vi "Day 6.vi"() -> ()   [LabVIEW 2020]
uses:
  3fa8e623-7fc4-4fee-bd88-71eac602b765.vi
  8efd2a67-bb32-401c-9d86-5bcad490fe8b.vi
panel:
  out "Solution":i32
  out "Solution":i32
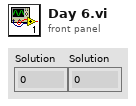
[diagram p1: front panel]
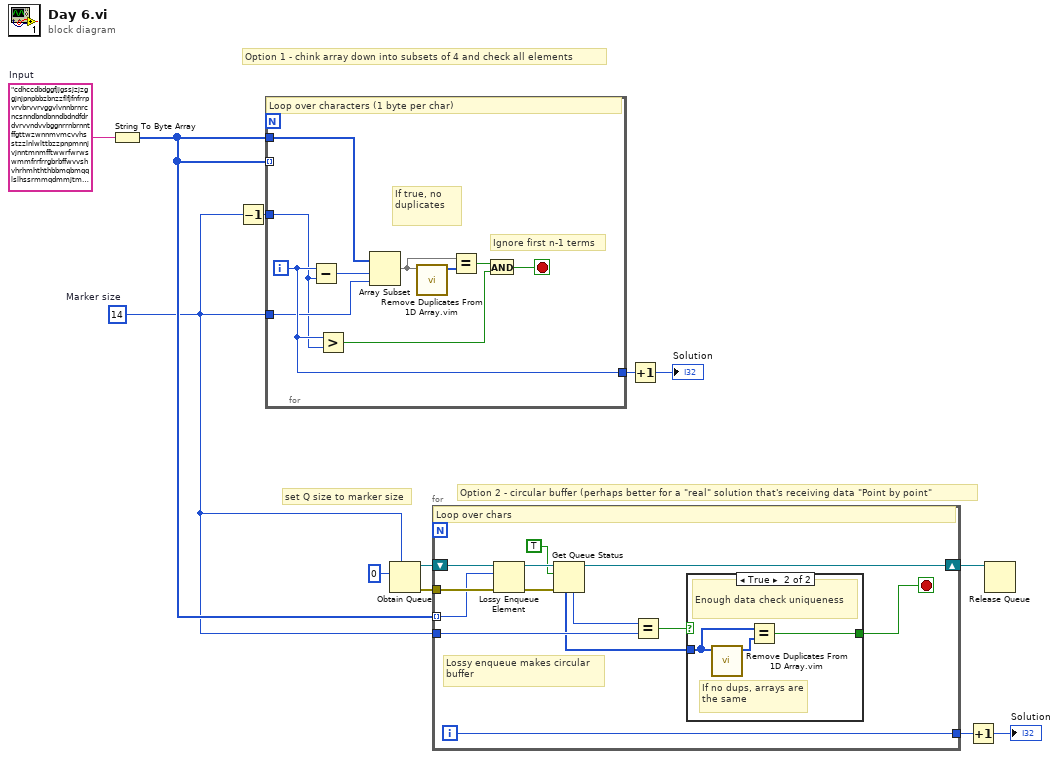
[diagram p0: block diagram]
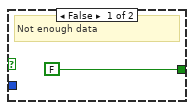
[diagram p2: hidden frame]
diagram:
  w5 = 14  # Marker size
  w9 = "cdhccdbdggfjjgssjzjzggjnjpnpbbzbnzzflfjfnfrrpvrvbrvvrvggvlvnnbrnrcncsnndbndbnndbdndfdrdvrvvndvvbggnrrnbrnntffgttwzwnnmvmcvvhsstzzlnlwlttbzzpnpmnnjvjnntmnmfftwwrfwrwswmmfrrfrrgbrbffwvvshvhrhmhththbbmqbmqqlslhssrmmqdmmjtmtmjtmjtttnwnvwvqwqjjnbbbdbqbnbpnbnllglcglcgcdczdznnqhhfthtmtlldqlqrrmddrldlzdllvddjcddqfqbqsbqqnllwppqpqzzrbbdppzsppjdpdqpdqdfqfrrwbwrwwqcqcsqsvvpbvbbztzptzzpccdtdhdffvqvcvzzmwzwddjfdffplplqlvlmmmvggpmpvpddpbptplpvlplvpvvnrvnnbqqqjhhwfhwfhwhqhmmpphqpqvppfzpzjzddgzzwffjmjggwhwwnnmlmpmmhcmcpcrcddvzvpzzwnznfznffgdgvddvtvgvsvdsdbbjnjtntbnttgbbbvgvgrgrzrvzrzddlsddcndcnnfqnnmpmlppdlpl..."  # Input
  # "Option 2 - circular buffer (perhaps better for a \"real\" solution that's receiving data \"Point by point\""
  # "Option 1 - chink array down into subsets of 4 and check all elements"
  # "set Q size to marker size"
  n1 = String To Byte Array(string=w9) -> (unsigned byte array=w8:u8[])
  n2 = Decrement(x=w5) -> (x-1=w10:i32)
  n3 = for {
    tunnel: w8 -> [w22]
    tunnel: [w20] -> w12
    tunnel: w5 -> [w17]
    tunnel: w10 -> [w16]
    tunnel: w8 -> [_] mode=indexing
    i -> [w20]
    stop <- w18 stop-if-true
    # "Ignore first n-1 terms"
    # "If true, no duplicates"
    # "Loop over characters (1 byte per char)"
    n4 = Subtract(x=w20, y=w16) -> (x-y=w21:i32)
    n5 = Greater?(x=w20, y=w16) -> (0:w19:bool)
    n6 = Array Subset(array=w22, index=w21, length=w17) -> (w14:u8[])
    n7 = call "Remove Duplicates From 1D Array.vim"("array"=w14) -> ("array with duplicates removed"=w15:u8[])  [unwired: 10 in]
    n8 = Equal?(x=w14, y=w15) -> (x = y?=w13:bool)
    n9 = And(x=w13, y=w19) -> (x .and. y?=w18:bool)
  }
  n10 = Obtain Queue(max queue size (-1, unlimited)=w5, element data type=u8 0) -> (queue out=w6:refnum<queue>, error out=w7:errorcluster)  [unwired: 3 in, 1 out]
  n11 = for {
    tunnel: w8 -> [w33] mode=indexing
    tunnel: w7 -> [w35]
    tunnel: w5 -> [w29]
    tunnel: [w24] -> w4
    shift-right: [w23] -> w1
    shift-left: w6 -> [w34]
    i -> [w24]
    stop <- w25 stop-if-true
    # "Lossy enqueue makes circular\nbuffer"
    # "Loop over chars"
    n12 = Lossy Enqueue Element(queue=w34, element=w33, error in (no error)=w35) -> (queue out=w31:refnum<queue>, error out=w32:errorcluster)  [unwired: 2 out]
    n13 = Get Queue Status(queue=w31, return elements? (F)=TRUE, error in (no error)=w32) -> (queue out=w23:refnum<queue>, # elements in queue=w28:i32, elements=w26:u8[])  [unwired: 5 out]
    n14 = Equal?(x=w28, y=w29) -> (x = y?=w27:bool)
    n15 = case shown="True" w27 {
      tunnel: w26 -> [_ w37]
      tunnel: [FALSE w38] -> w25
      frame False {
        # "Not enough data"
      }
      frame True {
        # "If no dups, arrays are the same"
        # "Enough data check uniqueness"
        n16 = call "Remove Duplicates From 1D Array.vim"("array"=w37) -> ("array with duplicates removed"=w39:u8[])  [unwired: 10 in]
        n17 = Equal?(x=w37, y=w39) -> (x = y?=w38:bool)
      }
    }
  }
  n18 = Increment(x=w12) -> (x+1=→"Solution":i32)
  n19 = Increment(x=w4) -> (x+1=→"Solution":i32)
  n20 = Release Queue(queue=w1) -> ()  [unwired: 2 in, 3 out]
